vi "LIA Simulation SOS.vi"() -> ()   [LabVIEW 2018]
uses:
  Shared/sos/Controls/iir_coefficients.ctl
  <instrlib>/_niInstr/DSP/v1/Shared/Public/IQ Data.ctl
  <vilib>/measure/maspectr.llb/FFT Power Spectrum and PSD for 1 Chan (CDB).vi
  <vilib>/Analysis/NI_AALBase.lvlib
  <vilib>/measure/NI_MAPro.lvlib
  <instrlib>/_niInstr/DSP/v1/Shared/niInstr DSP v1 Shared.lvlib
panel:
  out "size(s)":i32
  in  "Decimation (-1)":dbl=4.0 format="%#_p"
  out "Numeric":i32
  out "Waveform Graph 3":dbl[][](graph)
  out "Waveform Graph 2":cluster{"f0":dbl, "df":dbl, "magnitude":dbl[]}(graph)
  in  "IIR 2 coeffs":T1={"b0"=0.001556396484375, "b1"=-0.000762939453125, "-a1"=1.9305267333984375, "-a2"=-0.9328765869140625}
  out "Waveform Graph":cluster{"f0":dbl, "df":dbl, "magnitude":dbl[]}(graph)
  in  "Sampling Rate":dbl=1.0 format="%#_p"
  out "FFT Gain":dbl
  out "Noise (W|50ohms)":dbl
  out "k":dbl
  out "Noise vrms":dbl
  in  "Desired SNR (dB)":dbl format="%#_p"
  in  "Oscillator Magnitude":dbl=1.0 format="%#_13g"
  in  "Oscillator Frequency":dbl=0.001 format="%#_p"
  in  "Signal Offset":cdb format="%#_13g"
  in  "Singal Amplitude":dbl=0.5 format="%#_13g"
  in  "Signal Frequency":dbl=0.001 format="%#_p"
  in  "Number Samples":i32=10000
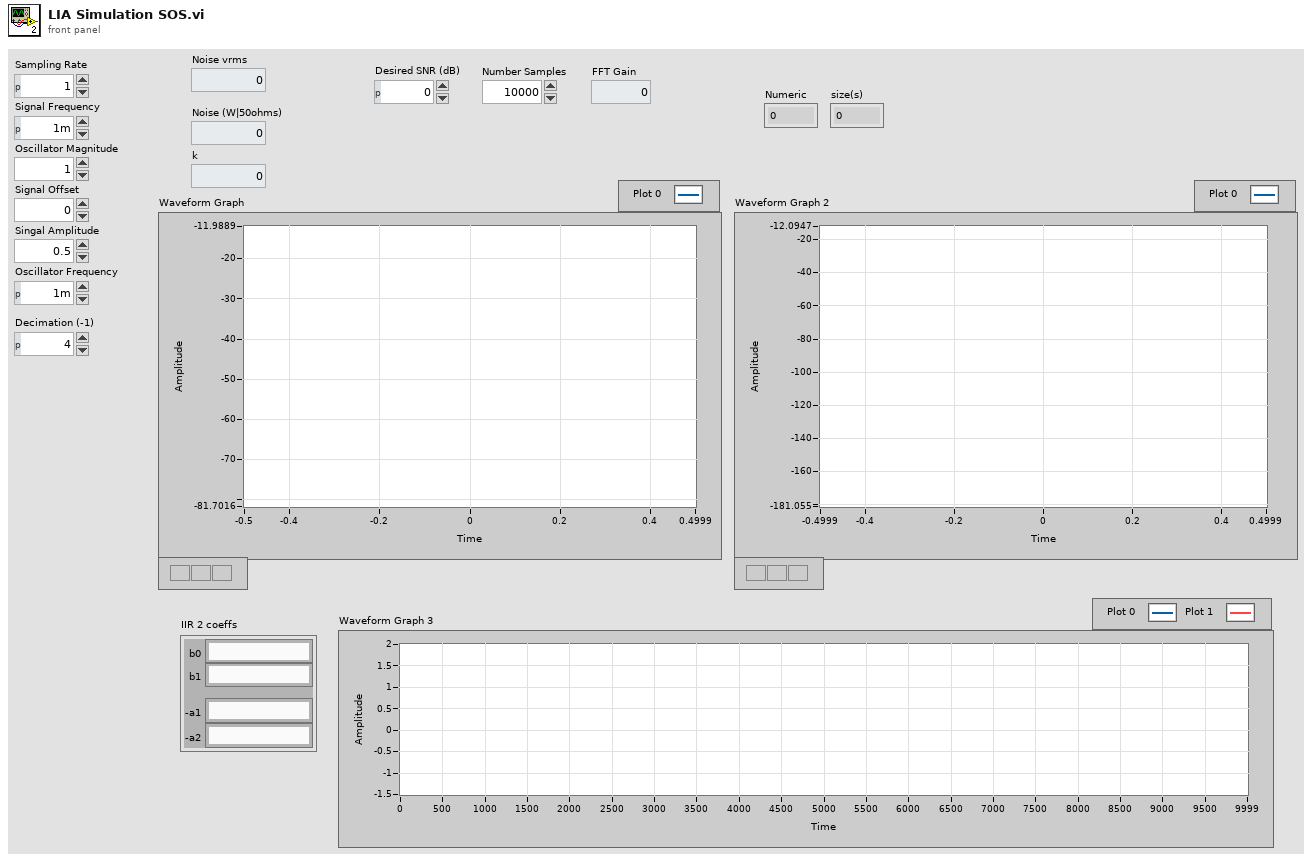
[diagram p1: front panel]
types:
  T1 = typedef "iir_coefficients.ctl" = cluster{"b0":fxp<+/-,18,2>, "b1":fxp<+/-,18,2>, "-a1":fxp<+/-,18,2>, "-a2":fxp<+/-,18,2>}
  T2 = typedef "niInstr DSP v1 Shared.lvlib/IQ Data.ctl" = cluster{"I":fxp<+/-,18,1>, "Q":fxp<+/-,18,1>, "overflow":bool}
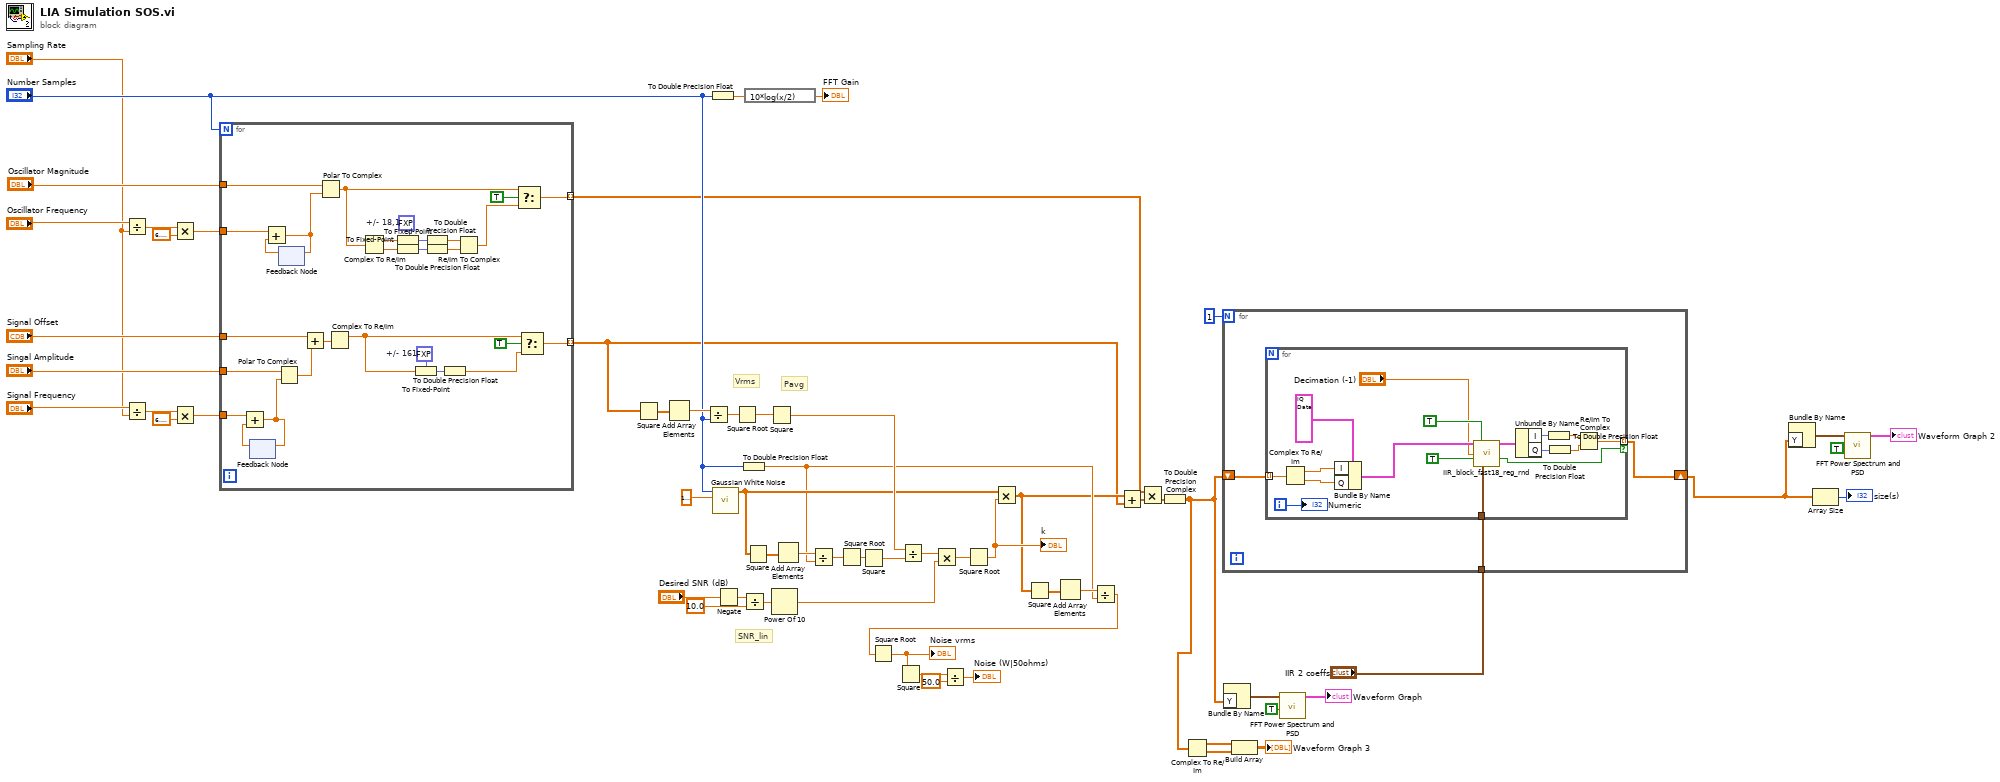
[diagram p0: block diagram]
diagram:
  # "SNR_lin"
  # "Pavg"
  # "Vrms"
  n1 = Divide(x="Oscillator Frequency", y="Sampling Rate") -> (x/y=w56:dbl)
  n2 = Divide(x="Signal Frequency", y="Sampling Rate") -> (x/y=w60:dbl)
  n3 = Multiply(x=w56, y=6.283185307179586) -> (x*y=w53:dbl)
  n4 = Multiply(x=w60, y=6.283185307179586) -> (x*y=w59:dbl)
  n5 = for {
    N: "Number Samples" -> [_]
    tunnel: w59 -> [w86]
    tunnel: "Singal Amplitude" -> [w89]
    tunnel: "Signal Offset" -> [w88]
    tunnel: [w72] -> w1 mode=indexing
    tunnel: [w66] -> w18 mode=indexing
    tunnel: w53 -> [w77]
    tunnel: "Oscillator Magnitude" -> [w75]
    w67 = fxp<+/-,16,1> 0.0  # +/- 161
    w82 = fxp<+/-,18,1> 0.0  # +/- 18,1
    n6 = feedback #1() -> (w90:dbl)  [unwired: 1 in]
    n7 = Add(x=w86, y=w90) -> (x+y=w85:dbl)
    n8 = feedback-in #1(w85) -> ()
    n9 = Polar To Complex(1:w85, 2:w89) -> (0:w87:cdb)
    n10 = feedback #2() -> (w76:dbl)  [unwired: 1 in]
    n11 = Add(x=w77, y=w76) -> (x+y=w74:dbl)
    n12 = feedback-in #2(w74) -> ()
    n13 = Add(x=w88, y=w87) -> (x+y=w64:cdb)
    n14 = Polar To Complex(1:w74, 2:w75) -> (0:w73:cdb)
    n15 = Complex To Re/Im(x + iy=w64) -> (x=w63:dbl)  [unwired: 1 out]
    n16 = Complex To Re/Im(x + iy=w73) -> (x=w84:dbl, y=w83:dbl)
    n17 = To Fixed-Point(fixed-point type=w82, number=w84) -> (fixed-point=w81:fxp<+/-,18,1>)
    n18 = To Fixed-Point(fixed-point type=w82, number=w83) -> (fixed-point=w80:fxp<+/-,18,1>)
    n19 = To Fixed-Point(fixed-point type=w67, number=w63) -> (fixed-point=w68:fxp<+/-,16,1>)
    n20 = To Double Precision Float(number=w81) -> (double precision float=w79:dbl)
    n21 = To Double Precision Float(number=w80) -> (double precision float=w78:dbl)
    n22 = To Double Precision Float(number=w68) -> (double precision float=w65:dbl)
    n23 = Re/Im To Complex(1:w78, 2:w79) -> (0:w71:cdb)
    n24 = Select(t=w73, s=TRUE, f=w71) -> (s? t:f=w72:cdb)
    n25 = Select(t=w63, s=TRUE, f=w65) -> (s? t:f=w66:dbl)
  }
  n26 = Square(x=w18) -> (x^2=w51:dbl[])
  n27 = Add Array Elements(numeric array=w51) -> (sum=w50:dbl)
  n28 = Divide(x=w50, y="Number Samples") -> (x/y=w49:dbl)
  n29 = To Double Precision Float(number="Number Samples") -> (double precision float=w23:dbl)
  n30 = call <vilib>:"Gaussian White Noise.vi"("standard deviation"=1.0000000000000002, "samples"="Number Samples") -> ("Gaussian noise pattern"=w33:dbl[])  [unwired: 8 in, 1 out]
  n31 = Negate(x="Desired SNR (dB)") -> (-x=w36:dbl)
  n32 = Square Root(x=w49) -> (sqrt(x)=w48:dbl)
  n33 = To Double Precision Float(number="Number Samples") -> (double precision float=w21:dbl)
  n34 = Divide(x=w36, y=10.0) -> (x/y=w44:dbl)
  n35 = expression code="10*log(x/2)"(w23) -> (→"FFT Gain":dbl)
  n36 = Square(x=w33) -> (x^2=w40:dbl[])
  n37 = Square(x=w48) -> (x^2=w39:dbl)
  n38 = Power Of 10(x=w44) -> (10^x=w35:dbl)
  n39 = Add Array Elements(numeric array=w40) -> (sum=w41:dbl)
  n40 = Divide(x=w41, y=w21) -> (x/y=w42:dbl)
  n41 = Square Root(x=w42) -> (sqrt(x)=w43:dbl)
  n42 = Square(x=w43) -> (x^2=w38:dbl)
  n43 = Divide(x=w39, y=w38) -> (x/y=w37:dbl)
  n44 = Multiply(x=w37, y=w35) -> (x*y=w34:dbl)
  n45 = Square Root(x=w34) -> (sqrt(x)=w32:dbl)
  "k" <- w32
  n46 = Multiply(x=w33, y=w32) -> (x*y=w19:dbl[])
  n47 = Square(x=w19) -> (x^2=w31:dbl[])
  n48 = Add Array Elements(numeric array=w31) -> (sum=w30:dbl)
  n49 = Divide(x=w30, y=w21) -> (x/y=w29:dbl)
  n50 = Square Root(x=w29) -> (sqrt(x)=w28:dbl)
  "Noise vrms" <- w28
  n51 = Square(x=w28) -> (x^2=w27:dbl)
  n52 = Divide(x=w27, y=50.0) -> (x/y=→"Noise (W|50ohms)":dbl)
  n53 = Add(x=w19, y=w18) -> (x+y=w17:dbl[])
  n54 = Multiply(x=w1, y=w17) -> (x*y=w2:cdb[])
  n55 = To Double Precision Complex(1:w2) -> (0:w9:cdb[])
  n56 = Complex To Re/Im(x + iy=w9) -> (x=w8:dbl[], y=w7:dbl[])
  n57 = for {
    N: 1 -> [_]
    tunnel: "IIR 2 coeffs" -> [w93]
    shift-right: [w91] -> w5
    shift-left: w9 -> [w92]
    n58 = for {
      tunnel: w92 -> [w108] mode=indexing
      tunnel: [w100] -> w91 mode=indexing if=w99
      tunnel: w93 -> [w98]
      i -> [w97]
      n59 = Complex To Re/Im(x + iy=w108) -> (x=w107:dbl, y=w106:dbl)
      n60 = Bundle By Name(cluster=T2 {"I"=0.0, "Q"=0.0, "overflow"=FALSE} ("IQ_Data_In"), "I"=w107, "Q"=w106) -> (w96:T2)
      n61 = call "IIR_block_fast18_reg_rnd.vi"("IQ_Data_In"=w96, "enable"=TRUE, "Decimation Factor (-1)"="Decimation (-1)", "Valid In"=TRUE, "IIR 2 coeffs"=w98) -> ("IQ_Data_Out"=w95:T2, "output valid"=w99:bool)  [unwired: 9 in]
      n62 = Unbundle By Name(w95) -> ("I"=w104:fxp<+/-,18,1>, "Q"=w103:fxp<+/-,18,1>)
      n63 = To Double Precision Float(number=w104) -> (double precision float=w102:dbl)
      n64 = To Double Precision Float(number=w103) -> (double precision float=w101:dbl)
      n65 = Re/Im To Complex(1:w101, 2:w102) -> (0:w100:cdb)
      "Numeric" <- w97
    }
  }
  n66 = Bundle By Name("Y"=w9) -> (w16:waveform(cdb))  [unwired: 1 in]
  n67 = Build Array(w8, w7) -> (→"Waveform Graph 3":dbl[][])
  n68 = call-poly <vilib>:"FFT Power Spectrum and PSD.vi"("dB On (F)"=TRUE, "time signal"=w16) -> ("Power Spectrum / PSD"=→"Waveform Graph":cluster{"f0":dbl, "df":dbl, "magnitude":dbl[]})  [unwired: 6 in, 3 out]
  n69 = Bundle By Name("Y"=w5) -> (w11:waveform(cdb))  [unwired: 1 in]
  n70 = Array Size(array=w5) -> (size(s)=→"size(s)":i32)
  n71 = call-poly <vilib>:"FFT Power Spectrum and PSD.vi"("dB On (F)"=TRUE, "time signal"=w11) -> ("Power Spectrum / PSD"=→"Waveform Graph 2":cluster{"f0":dbl, "df":dbl, "magnitude":dbl[]})  [unwired: 6 in, 3 out]
